vi "ConcatenateNonBlanks.vi"(1 "separator":string=";", 5 "prependString":string, 9 "appendString":string) -> (8 "outputString":string)   [LabVIEW 2016]
doc: "Concatenates strings, WITHOUT putting separators where the string are null or whitespace"
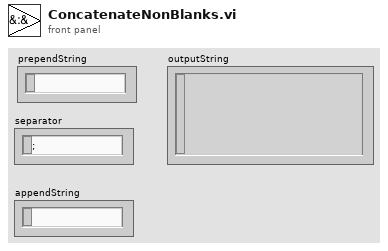
[diagram p1: front panel]
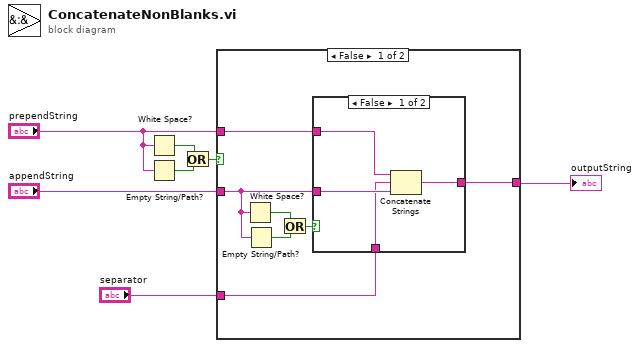
[diagram p0: block diagram]
diagram:
  n1 = White Space?(1:"prependString") -> (0:w5:bool)
  n2 = Empty String/Path?(string/path="prependString") -> (empty?=w1:bool)
  n3 = Or(x=w5, y=w1) -> (x .or. y?=w2:bool)
  n4 = case shown="False" w2 {
    tunnel: "appendString" -> [w10 w20]
    tunnel: [w14 w20] -> w7
    tunnel: "prependString" -> [w13 _]
    tunnel: "separator" -> [w12 _]
    frame False {
      n5 = White Space?(1:w10) -> (0:w9:bool)
      n6 = Empty String/Path?(string/path=w10) -> (empty?=w11:bool)
      n7 = Or(x=w9, y=w11) -> (x .or. y?=w8:bool)
      n8 = case shown="False" w8 {
        tunnel: w10 -> [w18 _]
        tunnel: [w17 w19] -> w14
        tunnel: w13 -> [w16 w19]
        tunnel: w12 -> [w15 _]
        frame False {
          n9 = Concatenate Strings(w16, w15, w18) -> (w17:string)
        }
        frame True {
        }
      }
    }
    frame True {
    }
  }
  "outputString" <- w7
